vi "Position_One_Scoring.vi"(11 "Stop":string) -> (3 "concatenated string":string)   [LabVIEW 2012, in "Serenity_mk2.lvrbt"]
uses:
  Serenity_mk2.lvrbt
  auto_drive_TYP.ctl
  State_Typ.ctl
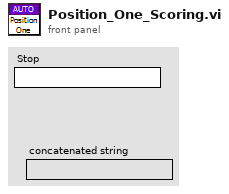
[diagram p1: front panel]
types:
  T1 = typedef "auto_drive_TYP.ctl" = cluster{"Left X":i8, "Left Y":i8, "Right Y":i8, "Power (100)":i8, "Wait (ms)":u32, "Enc/Deg Target":i32, "Move Type":enum16{"Relative Degrees", "Wait", "Encoder"}}
  T2 = typedef "State_Typ.ctl" = enum16{"Sweeper", "Stop", "Check for Position 3", "Check for Position 2", "Move", "Reset Enc", "Read Enc", "Lift", "Dump Close"}
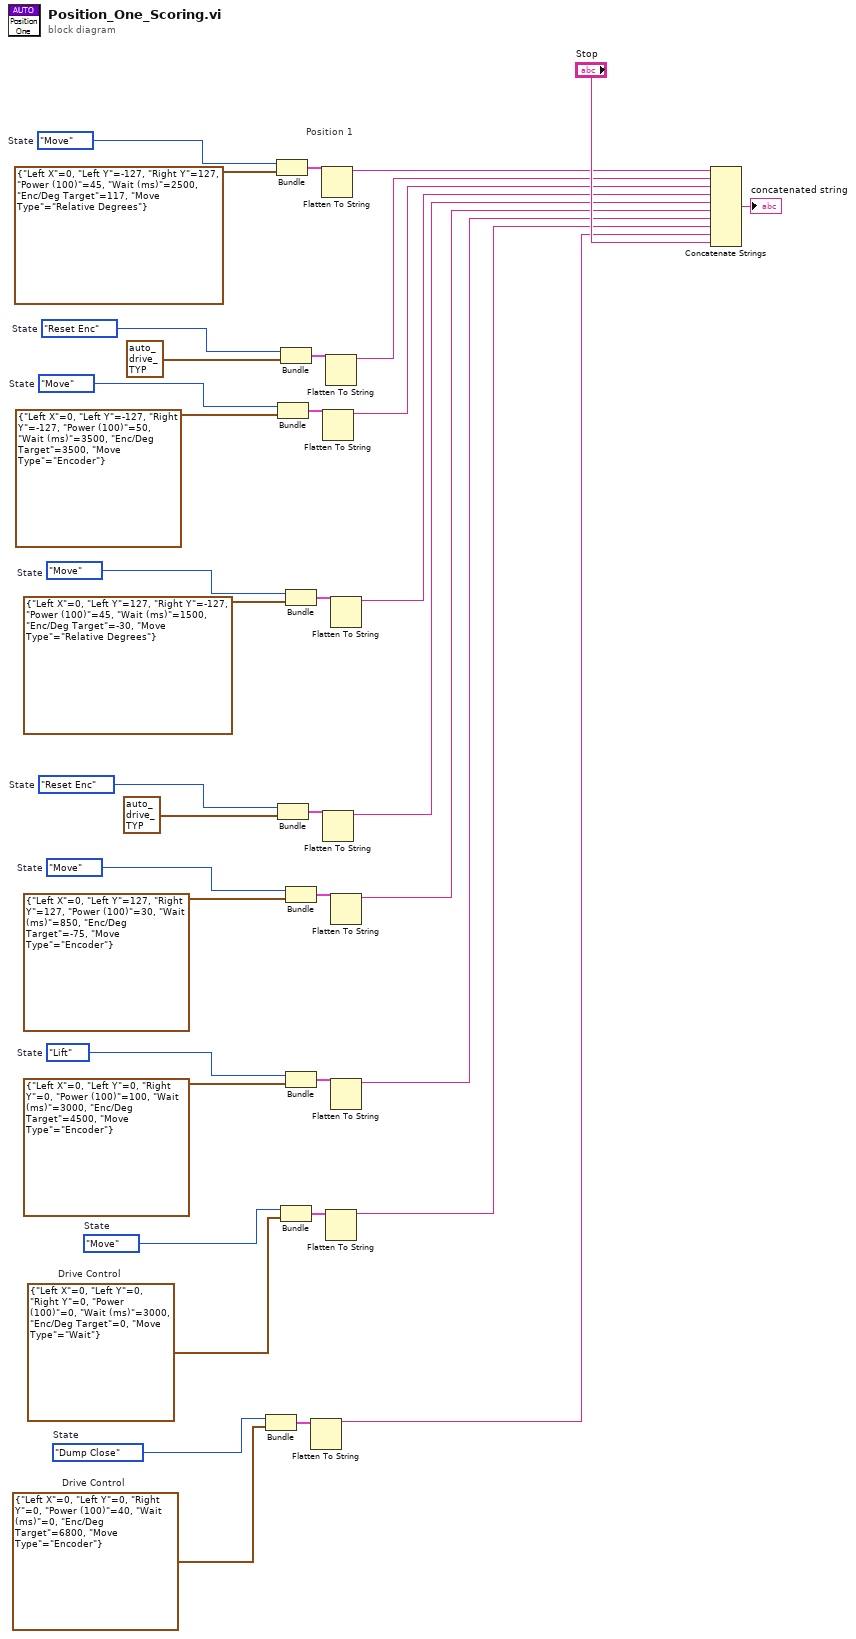
[diagram p0: block diagram]
diagram:
  w36 = State_Typ."Reset Enc"  # State
  w31 = T1 {"Left X"=0, "Left Y"=0, "Right Y"=0, "Power (100)"=40, "Wait (ms)"=0, "Enc/Deg Target"=6800, "Move Type"=enum."Encoder"}  # Drive Control
  w30 = State_Typ."Dump Close"  # State
  w28 = T1 {"Left X"=0, "Left Y"=0, "Right Y"=0, "Power (100)"=0, "Wait (ms)"=3000, "Enc/Deg Target"=0, "Move Type"=enum."Wait"}  # Drive Control
  w27 = State_Typ."Move"  # State
  w26 = State_Typ."Move"  # State
  w21 = State_Typ."Lift"  # State
  w19 = State_Typ."Move"  # State
  w15 = State_Typ."Reset Enc"  # State
  w9 = State_Typ."Move"  # State
  w7 = State_Typ."Move"  # State
  # "Position 1"
  n1 = Bundle("State"=w30, "Drive Control"=w31) -> (w32:cluster{"State":T2, "Drive Control":T1})  [unwired: 1 in]
  n2 = Bundle("State"=w7, "Drive Control"=T1 {"Left X"=0, "Left Y"=-127, "Right Y"=127, "Power (100)"=45, "Wait (ms)"=2500, "Enc/Deg Target"=117, "Move Type"=enum."Relative Degrees"}) -> (w6:cluster{"State":T2, "Drive Control":T1})  [unwired: 1 in]
  n3 = Bundle("State"=w9, "Drive Control"=T1 {"Left X"=0, "Left Y"=-127, "Right Y"=-127, "Power (100)"=50, "Wait (ms)"=3500, "Enc/Deg Target"=3500, "Move Type"=enum."Encoder"}) -> (w10:cluster{"State":T2, "Drive Control":T1})  [unwired: 1 in]
  n4 = Bundle("State"=w36, "Drive Control"=T1 {"Left X"=0, "Left Y"=127, "Right Y"=127, "Power (100)"=50, "Wait (ms)"=4000, "Enc/Deg Target"=-136, "Move Type"=enum."Relative Degrees"}) -> (w35:cluster{"State":T2, "Drive Control":T1})  [unwired: 1 in]
  n5 = Bundle("State"=w15, "Drive Control"=T1 {"Left X"=0, "Left Y"=127, "Right Y"=127, "Power (100)"=50, "Wait (ms)"=4000, "Enc/Deg Target"=-136, "Move Type"=enum."Relative Degrees"}) -> (w14:cluster{"State":T2, "Drive Control":T1})  [unwired: 1 in]
  n6 = Bundle("State"=w27, "Drive Control"=w28) -> (w29:cluster{"State":T2, "Drive Control":T1})  [unwired: 1 in]
  n7 = Bundle("State"=w19, "Drive Control"=T1 {"Left X"=0, "Left Y"=127, "Right Y"=-127, "Power (100)"=45, "Wait (ms)"=1500, "Enc/Deg Target"=-30, "Move Type"=enum."Relative Degrees"}) -> (w18:cluster{"State":T2, "Drive Control":T1})  [unwired: 1 in]
  n8 = Bundle("State"=w26, "Drive Control"=T1 {"Left X"=0, "Left Y"=127, "Right Y"=127, "Power (100)"=30, "Wait (ms)"=850, "Enc/Deg Target"=-75, "Move Type"=enum."Encoder"}) -> (w24:cluster{"State":T2, "Drive Control":T1})  [unwired: 1 in]
  n9 = Bundle("State"=w21, "Drive Control"=T1 {"Left X"=0, "Left Y"=0, "Right Y"=0, "Power (100)"=100, "Wait (ms)"=3000, "Enc/Deg Target"=4500, "Move Type"=enum."Encoder"}) -> (w22:cluster{"State":T2, "Drive Control":T1})  [unwired: 1 in]
  n10 = Flatten To String(anything=w32) -> (data string=w33:string)  [unwired: 3 in, 2 out]
  n11 = Flatten To String(anything=w6) -> (data string=w8:string)  [unwired: 3 in, 2 out]
  n12 = Flatten To String(anything=w10) -> (data string=w12:string)  [unwired: 3 in, 2 out]
  n13 = Flatten To String(anything=w35) -> (data string=w37:string)  [unwired: 3 in, 2 out]
  n14 = Flatten To String(anything=w14) -> (data string=w16:string)  [unwired: 3 in, 2 out]
  n15 = Flatten To String(anything=w29) -> (data string=w3:string)  [unwired: 3 in, 2 out]
  n16 = Flatten To String(anything=w18) -> (data string=w20:string)  [unwired: 3 in, 2 out]
  n17 = Flatten To String(anything=w24) -> (data string=w2:string)  [unwired: 3 in, 2 out]
  n18 = Flatten To String(anything=w22) -> (data string=w1:string)  [unwired: 3 in, 2 out]
  n19 = Concatenate Strings(w8, w16, w12, w20, w37, w2, w1, w3, w33, "Stop") -> (→"concatenated string":string)
